vi "All of the Lift.vi"(7 "Speed":dbl=0.25, 11 "Inches to move":dbl) -> (2 "Done":bool)   [LabVIEW 2014]
uses:
  Global Variables.vi
panel:
  in  "constant":dbl=200.0
  in  "right PID gains":T1={"proportional gain (Kc)"=0.006, "integral time (Ti, min)"=0.0, "derivative time (Td, min)"=0.0} {"derivative time (Td, min)" format="%.4f"; "integral time (Ti, min)" format="%.6f"; "proportional gain (Kc)" format="%.5f"}
  in  "left PID gains":T2={"proportional gain (Kc)"=0.006, "integral time (Ti, min)"=0.0, "derivative time (Td, min)"=0.0005} {"derivative time (Td, min)" format="%.10f"; "proportional gain (Kc)" format="%.5f"}
  in  "Output Range":cluster{"output high":dbl, "output low":dbl}={"output high"=0.5, "output low"=-0.5} {"output low" format="%.2f"; "output high" format="%.2f"}
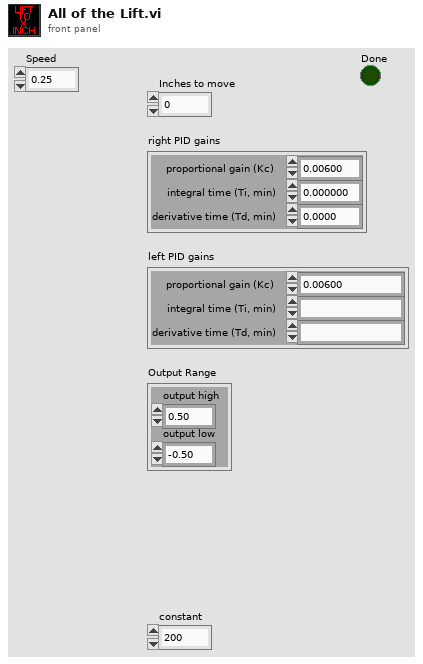
[diagram p1: front panel]
types:
  T1 = cluster{"proportional gain (Kc)":dbl, "integral time (Ti, min)":dbl, "derivative time (Td, min)":dbl}
  T2 = cluster{"proportional gain (Kc)":dbl, "integral time (Ti, min)":fxp<+/-,64,32>, "derivative time (Td, min)":dbl}
  T3 = typedef "WPI_EncoderDevRef.ctl" = cluster{"DevStatus":errorcluster, "EncoderIndex":T4, "CounterIndex":T5, "DistancePerCount":dbl, "Decoding Type":T6}
  T4 = typedef "FPGA_EncoderIdx.ctl" = enum8{"Enc 0", "Enc 1", "Enc 2", "Enc 3", "Enc 4", "Enc 5", "Enc 6", "Enc 7", "Invalid"}
  T5 = typedef "FPGA_CounterCtrSystemIndex.ctl" = enum8{"Ctr 0", "Ctr 1", "Ctr 2", "Ctr 3", "Ctr 4", "Ctr 5", "Ctr 6", "Ctr 7", "Invalid"}
  T6 = typedef "WPI_EncoderType.ctl" = enum16{"1x", "2x", "4x"}
  T7 = typedef "WPI_MotorControlDeviceRef.ctl" = cluster{"DeviceStatus":errorcluster, "Type":T8, "PWM":cluster{"Controller":T9, "PWM Channel":T10, "DeadBand":T11}, "CAN":cluster{"Device Number":u8, "Control Mode":T12, "Semaphore":T13, "Max Vout":dbl, "TalonSRX Control Mode":T14}, "Invert":bool, "TransformRef":T15, "InvTransformRef":T15}
  T8 = typedef "WPI_MotorControlType.ctl" = enum16{"PWM", "CAN", "CANTalonSRX"}
  T9 = typedef "FPGA_TypedefDigitalModule.ctl" = enum16{"Controller 1"}
  T10 = typedef "FPGA_DIOPWMChannel.ctl" = enum8{"PWM 0", "PWM 1", "PWM 2", "PWM 3", "PWM 4", "PWM 5", "PWM 6", "PWM 7", "PWM 8", "PWM 9", "PWM MXP 0", "PWM MXP 1", "PWM MXP 2", "PWM MXP 3", "PWM MXP 4", "PWM MXP 5", "PWM MXP 6", "PWM MXP 7", "PWM MXP 8", "PWM MXP 9", "Invalid"}
  T11 = typedef "WPI_PWMDeadband.ctl" = cluster{"Name":string, "maxPositivePwm":i32, "minPositivePwm":i32, "centerPwm":i32, "maxNegativePwm":i32, "minNegativePwm":i32, "angularRange":u16}
  T12 = typedef "WPI_CANJaguar_ControlMode.ctl" = enum8{"Percent VBus", "Current", "Speed", "Position", "Voltage"}
  T13 = typedef "Semaphore RefNum" = refnum<k1>
  T14 = typedef "WPI_CANTalonSRX_APIControlMode.ctl" = enum8{"Percent VBus", "Speed", "Position", "Slave", "Unchanged / Invalid"}
  T15 = typedef "WPI_PWMTransform_ConPane.ctl" = refnum<vi>
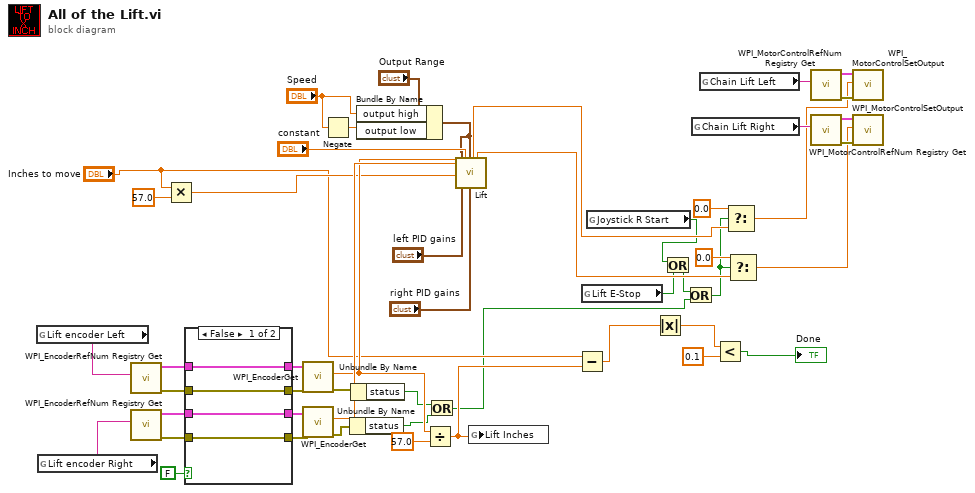
[diagram p0: block diagram]
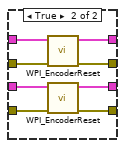
[diagram p2: hidden frame]
diagram:
  n1 = global read "Global Variables.vi" "Lift encoder Left"() -> (w44:string)
  n2 = global read "Global Variables.vi" "Lift encoder Right"() -> (w45:string)
  n3 = call <vilib>:"WPI_EncoderRefNum Registry Get.vi"("refnum name"=w44) -> ("error out"=w43:errorcluster, "EncoderDevRef"=w42:T3)  [unwired: 9 in]
  n4 = call <vilib>:"WPI_EncoderRefNum Registry Get.vi"("refnum name"=w45) -> ("error out"=w40:errorcluster, "EncoderDevRef"=w41:T3)  [unwired: 9 in]
  n5 = Multiply(x="Inches to move", y=57.0) -> (x*y=w23:dbl)
  n6 = case shown="False" FALSE {
    tunnel: w40 -> [w51 w62]
    tunnel: w41 -> [w52 w61]
    tunnel: w43 -> [w53 w59]
    tunnel: w42 -> [w54 w60]
    tunnel: [w54 w58] -> w47
    tunnel: [w52 w57] -> w48
    tunnel: [w51 w56] -> w49
    tunnel: [w53 w55] -> w50
    frame False {
    }
    frame True {
      n7 = call <vilib>:"WPI_EncoderReset.vi"("error in (no error)"=w59, "EncoderDevRef"=w60) -> ("error out"=w55:errorcluster, "EncoderDevRef"=w58:T3)  [unwired: 8 in]
      n8 = call <vilib>:"WPI_EncoderReset.vi"("error in (no error)"=w62, "EncoderDevRef"=w61) -> ("error out"=w56:errorcluster, "EncoderDevRef"=w57:T3)  [unwired: 8 in]
    }
  }
  n9 = call <vilib>:"WPI_EncoderGet.vi"("error in (no error)"=w50, "EncoderDevRef"=w47) -> ("error out"=w7:errorcluster, "Distance"=w28:dbl)  [unwired: 4 in, 4 out]
  n10 = call <vilib>:"WPI_EncoderGet.vi"("error in (no error)"=w49, "EncoderDevRef"=w48) -> ("error out"=w4:errorcluster, "Distance"=w37:dbl)  [unwired: 4 in, 4 out]
  n11 = Negate(x="Speed") -> (-x=w25:dbl)
  n12 = Unbundle By Name(w4) -> ("status"=w3:bool)
  n13 = Unbundle By Name(w7) -> ("status"=w5:bool)
  n14 = Bundle By Name(cluster="Output Range", "output high"="Speed", "output low"=w25) -> (w26:cluster{"output high":dbl, "output low":dbl})
  n15 = Divide(x=w28, y=57.0) -> (x/y=w22:dbl)
  n16 = Or(x=w5, y=w3) -> (x .or. y?=w2:bool)
  n17 = call "Lift.vi"("left encoder"=w28, "right encoder"=w37, "move to distance"=w23, "left output range"=w26, "left PID gains"="left PID gains", "constant"="constant", "right output range"=w26, "right PID gains"="right PID gains") -> ("lift motor left"=w10:dbl, "lift motor right"=w11:dbl)  [unwired: 18 in]
  n18 = global write "Global Variables.vi" "Lift Inches"(w22) -> ()
  n19 = Subtract(x="Inches to move", y=w22) -> (x-y=w21:dbl)
  n20 = global read "Global Variables.vi" "Lift E-Stop"() -> (w8:bool)
  n21 = global read "Global Variables.vi" "Joystick R Start"() -> (w9:bool)
  n22 = Absolute Value(x=w21) -> (abs(x)=w20:dbl)
  n23 = Or(x=w9, y=w8) -> (x .or. y?=w1:bool)
  n24 = Or(x=w1, y=w2) -> (x .or. y?=w6:bool)
  n25 = global read "Global Variables.vi" "Chain Lift Right"() -> (w33:string)
  n26 = global read "Global Variables.vi" "Chain Lift Left"() -> (w34:string)
  n27 = Less?(x=w20, y=0.1) -> (x < y?=→"Done":bool)
  n28 = Select(t=0.0, s=w6, f=w10) -> (s? t:f=w13:dbl)
  n29 = Select(t=0.0, s=w6, f=w11) -> (s? t:f=w12:dbl)
  n30 = call <vilib>:"WPI_MotorControlRefNum Registry Get.vi"("refnum name"=w34) -> ("error out"=w36:errorcluster, "MotorControlDevRef"=w35:T7)  [unwired: 9 in]
  n31 = call <vilib>:"WPI_MotorControlRefNum Registry Get.vi"("refnum name"=w33) -> ("error out"=w31:errorcluster, "MotorControlDevRef"=w32:T7)  [unwired: 9 in]
  n32 = call <vilib>:"WPI_MotorControlSetOutput.vi"("error in (no error)"=w36, "Output"=w13, "MotorControlDevRef"=w35) -> ()  [unwired: 6 in, 3 out]
  n33 = call <vilib>:"WPI_MotorControlSetOutput.vi"("error in (no error)"=w31, "Output"=w12, "MotorControlDevRef"=w32) -> ()  [unwired: 6 in, 3 out]
